vi "Update Offset Dialog.vi"(8 "error in":errorcluster, 10 "Test Result In":T2, 11 "CalCfg File In":T1) -> (0 "error out":errorcluster, 1 "Pass":bool, 2 "Test Result Out":T2, 3 "CalCfg File Out":T1, 4 "String":string)   [LabVIEW 2020, in "GUCalibration2.lvlib"]
uses:
  GUCalibration2.lvlib
  Controls/Test Result.ctl
  Controls/Site Data Element.ctl
  Controls/Site Raw Data Element.ctl
  Controls/Config Data Type.ctl
panel:
  in  "Export Table To CSV":bool
  out "GU Pass Count":string
  out "Result Table":string[][](table)=[["Site_1", "100101", "OS_PS_VDD1_ChA", "0.5", "mA", "0.455881", "0.00", "0.1", "0.2", "0.3", "0.022", ""], ["Site_1", "100102", "OS_PS_VDD1_ChB", "0.5", "uA", "0.467813", "0.00", "0.1", "0.2", "0.3", "0.1317", ""], ["Site_1", "100103", "OS_PS_VDD2_ChB", "0.5", "A", "0.448013", "0.00", "0.1", "0.2", "0.3", "0.0619", ""], ["Site_1", "100104", "OS_PS_SWVDD_ChAB", "0.5", "A", "0.437713", "0.00", "0.1", "0.2", "0.3", "-0.0484", ""], ["Site_1", "100105", "OS_VSS_PPMU_SWCTRL_ChAB", "-0.6", "V", "-0.52606", "0.00", "0.1", "0.2", "0.3", "0.0028", ""], ["Site_1", "100106", "OS_VSS_PPMU_PD_ChAB", "-0.6", "V", "-0.56283", "0.00", "0.1", "0.2", "0.3", "0.0016", ""], ["Site_1", "100107", "OS_VSS_PPMU_BP_ChA", "-0.6", "V", "-0.559845", "0.00", "0.1", "0.2", "0.3", "-0.0132", ""], ["Site_1", "100108", "OS_VSS_PPMU_BP_ChB", "-0.6", "V", "-0.559845", "0.00", "0.1", "0.2", "0.3", "-0.0632", ""], ["Site_1", "200101", "TX_SW_1V8_PD_1V8_BP_0_SWVDD1_ChAB", "0.3", "A", "0.316384", "0.00", "0.1", "0.2", "0.3", "-0.0241", ""], ["Site_1", "200102", "TX_SW_1V8_PD_1V8_BP_0_VDD1_ChA", "0.3", "A", "0.323078", "0.00", "0.1", "0.2", "0.3", "-0.0736", ""], ["Site_1", "200103", "TX_SW_1V8_PD_1V8_BP_0_VDD1_ChB", "0.3", "A", "0.316384", "0.00", "0.1", "0.2", "0.3", "-0.0741", ""], ["Site_1", "200104", "TX_SW_1V8_PD_1V8_BP_0_VDD2_ChB", "0.3", "A", "0.22866", "0.00", "0.1", "0.2", "0.3", "0.0354", ""], ["Site_1", "200105", "RX_SW_0_PD_0_BP_0_VDD1_ChA", "1.85", "A", "1.918991", "0.00", "0.1", "0.2", "0.5", "-0.0378", ""], ["Site_1", "200106", "RX_SW_0_PD_0_BP_0_VDD1_ChB", "1.85", "A", "1.918991", "0.00", "0.1", "0.2", "0.5", "-0.0678", ""], ["Site_1", "200107", "RX_SW_0_PD_0_BP_0_VDD2_ChB", "1.85", "A", "1.908841", "0.00", "0.1", "0.2", "0.5", "0.002", ""], ["Site_1", "200108", "RX_SW_0_PD_0_BP_0_SWVDD_ChAB", "1.85", "A", "1.980908", "0.00", "0.1", "0.2", "0.5", "-0.0686", ""], ["Site_0", "100101", "OS_PS_VDD1_ChA", "0.5", "mA", "0.412485", "0.00", "0.1", "0.2", "0.3", "-0.0147", ""], ["Site_0", "100102", "OS_PS_VDD1_ChB", "0.5", "uA", "0.492041", "0.00", "0.1", "0.2", "0.3", "0.0654", ""], ["Site_0", "100103", "OS_PS_VDD2_ChB", "0.5", "A", "0.481841", "0.00", "0.1", "0.2", "0.3", "0.0052", ""], ["Site_0", "100104", "OS_PS_SWVDD_ChAB", "0.5", "A", "0.471841", "0.00", "0.1", "0.2", "0.3", "-0.1048", ""], ["Site_0", "100105", "OS_VSS_PPMU_SWCTRL_ChAB", "-0.6", "V", "-0.636918", "0.00", "0.1", "0.2", "0.3", "-0.0902", ""], ["Site_0", "100106", "OS_VSS_PPMU_PD_ChAB", "-0.6", "V", "-0.706583", "0.00", "0.1", "0.2", "0.3", "-0.036", ""], ["Site_0", "100107", "OS_VSS_PPMU_BP_ChA", "-0.6", "V", "-0.744575", "0.00", "0.1", "0.2", "0.3", "-0.0387", ""], ["Site_0", "100108", "OS_VSS_PPMU_BP_ChB", "-0.6", "V", "-0.715075", "0.00", "0.1", "0.2", "0.3", "-0.0592", ""], ["Site_0", "200101", "TX_SW_1V8_PD_1V8_BP_0_SWVDD1_ChAB", "0.3", "A", "0.355752", "0.00", "0.1", "0.2", "0.3", "0.0175", ""], ["Site_0", "200102", "TX_SW_1V8_PD_1V8_BP_0_VDD1_ChA", "0.3", "A", "0.363553", "0.00", "0.1", "0.2", "0.3", "-0.03", ""], ["Site_0", "200103", "TX_SW_1V8_PD_1V8_BP_0_VDD1_ChB", "0.3", "A", "0.248228", "0.00", "0.1", "0.2", "0.3", "-0.0428", ""], ["Site_0", "200104", "TX_SW_1V8_PD_1V8_BP_0_VDD2_ChB", "0.3", "A", "0.237628", "0.00", "0.1", "0.2", "0.3", "0.0466", ""], ["Site_0", "200105", "RX_SW_0_PD_0_BP_0_VDD1_ChA", "1.85", "A", "1.71837", "0.00", "0.1", "0.2", "0.5", "0.0158", ""], ["Site_0", "200106", "RX_SW_0_PD_0_BP_0_VDD1_ChB", "1.85", "A", "1.71837", "0.00", "0.1", "0.2", "0.5", "-0.0142", ""], ["Site_0", "200107", "RX_SW_0_PD_0_BP_0_VDD2_ChB", "1.85", "A", "1.75781", "0.00", "0.1", "0.2", "0.5", "0.0696", ""], ["Site_0", "200108", "RX_SW_0_PD_0_BP_0_SWVDD_ChAB", "1.85", "A", "1.591898", "0.00", "0.1", "0.2", "0.5", "-0.1017", ""]]
  out "Update Execute?":bool
  out "Info Disp":string
  in  "Update Offset":bool
  in  "Cancel":bool
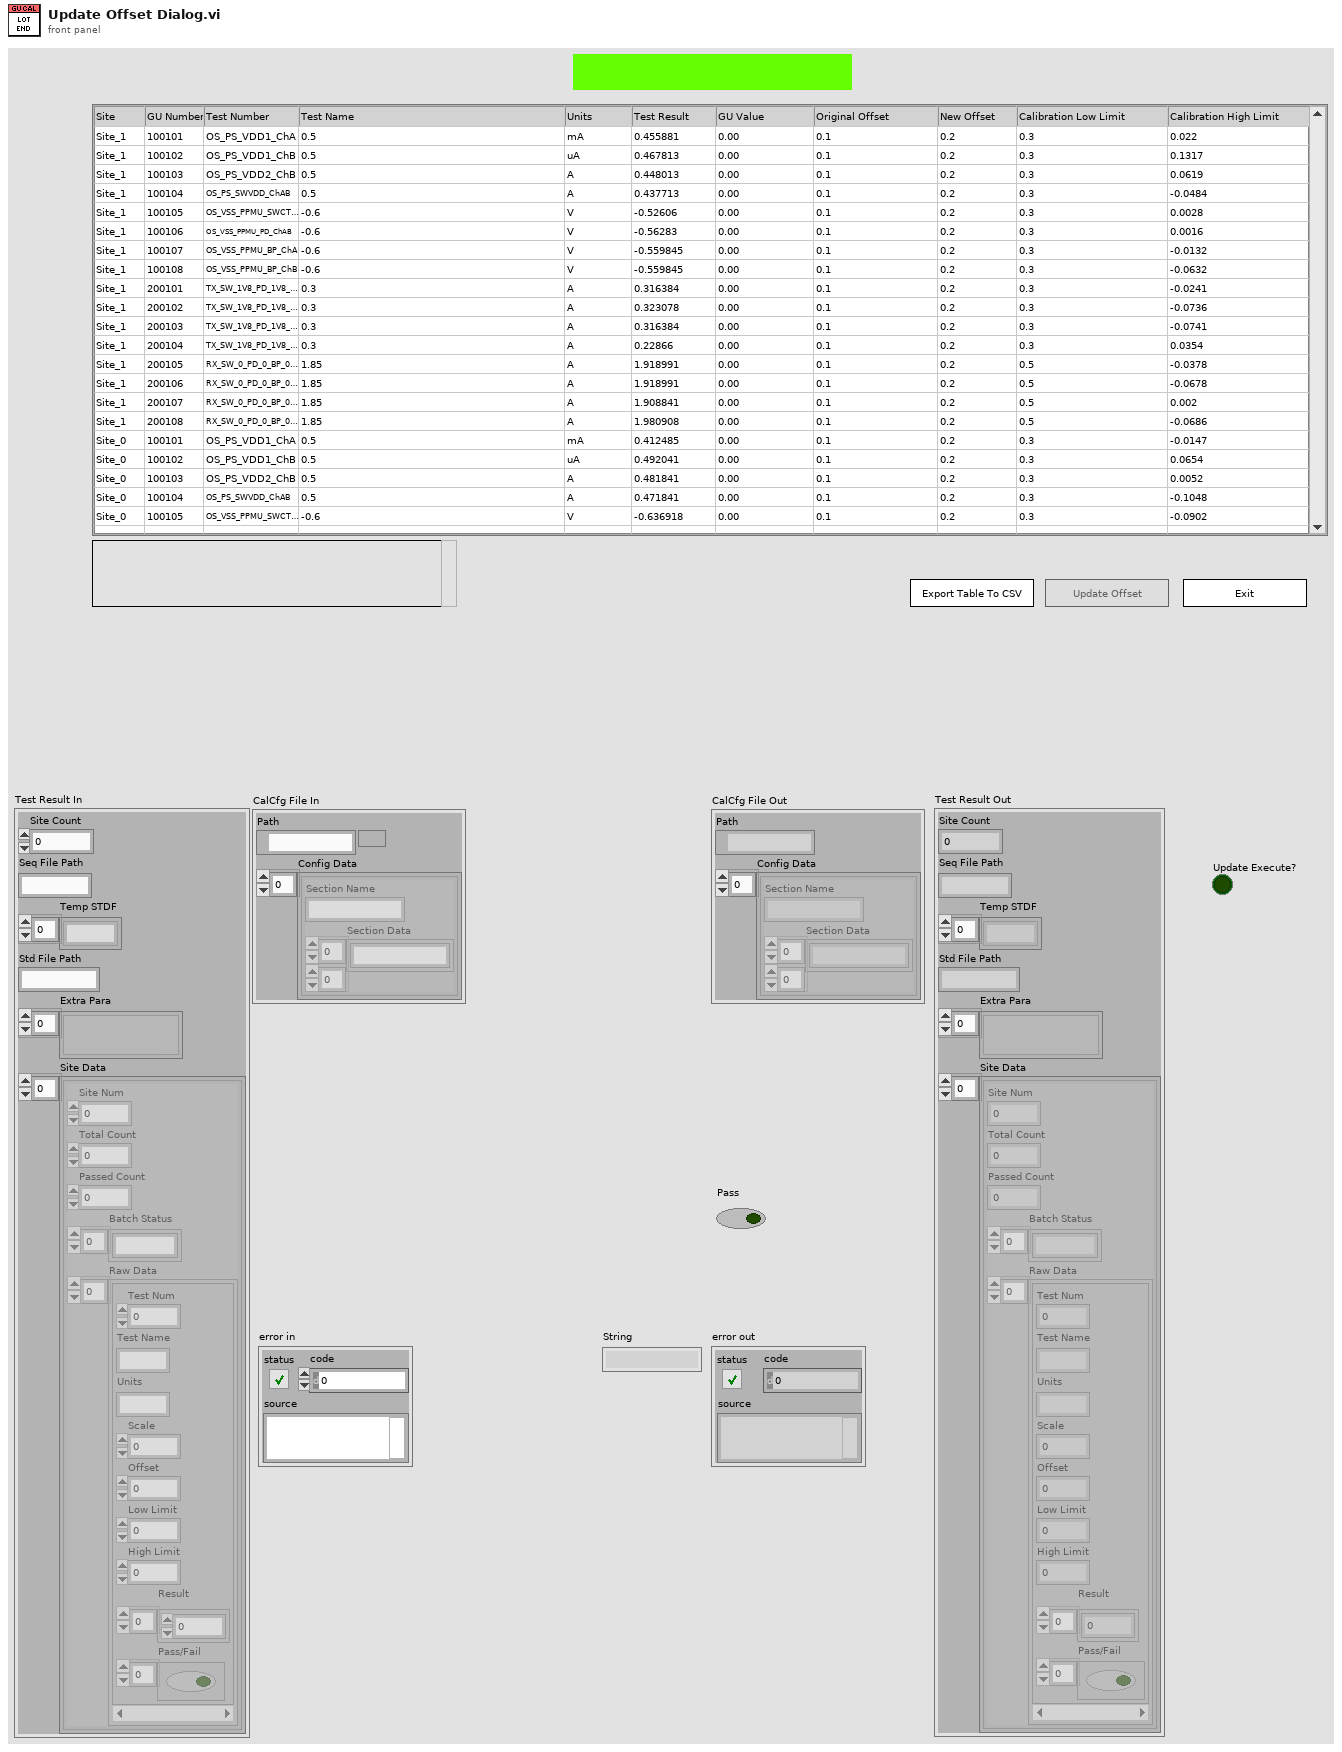
[diagram p1: front panel]
types:
  T1 = cluster{"Path":path, "Config Data":cluster{"Section Name":string, "Section Data":string[][]}[]}
  T2 = typedef "GUCalibration2.lvlib/Test Result.ctl" = cluster{"Site Count":i32, "Seq File Path":string, "Temp STDF":string[], "Std File Path":string, "Extra Para":variant[], "Site Data":T3[]}
  T3 = typedef "GUCalibration2.lvlib/Site Data Element.ctl" = cluster{"Site Num":i32, "Total Count":i32, "Passed Count":i32, "Batch Status":string[], "Raw Data":T4[]}
  T4 = typedef "GUCalibration2.lvlib/Site Raw Data Element.ctl" = cluster{"Test Num":u32, "Test Name":string, "Units":string, "Scale":i8, "Offset":dbl, "Low Limit":dbl, "High Limit":dbl, "Result":dbl[], "Pass/Fail":bool[]}
  T5 = typedef "GUCalibration2.lvlib/Config Data Type.ctl" = cluster{"Cal Type":i32, "Curr Batch Index":i32, "Loop Count Per GU":i32, "Min Num of Pass GUs Per Site":i32, "Is Calibration":bool, "Batch Iteration Done":bool, "Cal Abort":bool, "Update Offset":bool, "Cal Check Pass":bool, "Cal End":bool, "Enabled Site":i32[], "GU Selected":i32[], "All Available GU":i32[], "GU Arrange":i32[][], "Batch Test Count":i32[][], "Batch Test Result":string[][], "Curr Batch":i32[], "Curr Batch Test Count":i32[], "Curr Batch Target Count":i32[], "Curr Batch Test Result":string[]}
  T6 = cluster{"Result Table":refnum<vi>, "Error":errorcluster, "Exit":bool, "CorrOffset File":cluster{"File Path":path, "Backup File Path":path, "Offset Data":cluster{"Section Name":string, "Section Data":string[][]}[]}, "Calibration Cfg File":cluster{"Path":path, "Config Data":cluster{"Section Name":string, "Section Data":string[][]}[]}, "Test Result":T2, "Col Header":string[], "Data":string[][], "Update OK":bool, "Click Update":bool, "Limit Status":cluster{"Check Limit":bool[], "Cal Limit":bool[], "Cal GU Pass":bool[][], "Check GU Pass":bool[][], "Site Num":i32[], "GU Num":string[][]}, "IsCalibration":bool, "Info Disp":refnum<vi>, "CalType":i32, "Return String":string, "Final Offset":cluster{"Offset Info":cluster{"Site Number":string, "Test Number":string, "Units":string}[][], "Offset Value":string[][]}, "Cal Runtime Cfg":T5, "GU Pass Count Disp":refnum<vi>}
  T7 = cluster{"Section Name":string, "Section Data":string[][]}[]
  T8 = enum8{"Enabled", "Disabled", "Disabled and Grayed Out"}
  T9 = cluster{"File Path":path, "Backup File Path":path, "Offset Data":cluster{"Section Name":string, "Section Data":string[][]}[]}
  T10 = cluster{"Check Limit":bool[], "Cal Limit":bool[], "Cal GU Pass":bool[][], "Check GU Pass":bool[][], "Site Num":i32[], "GU Num":string[][]}
  T11 = cluster{"Offset Info":cluster{"Site Number":string, "Test Number":string, "Units":string}[][], "Offset Value":string[][]}
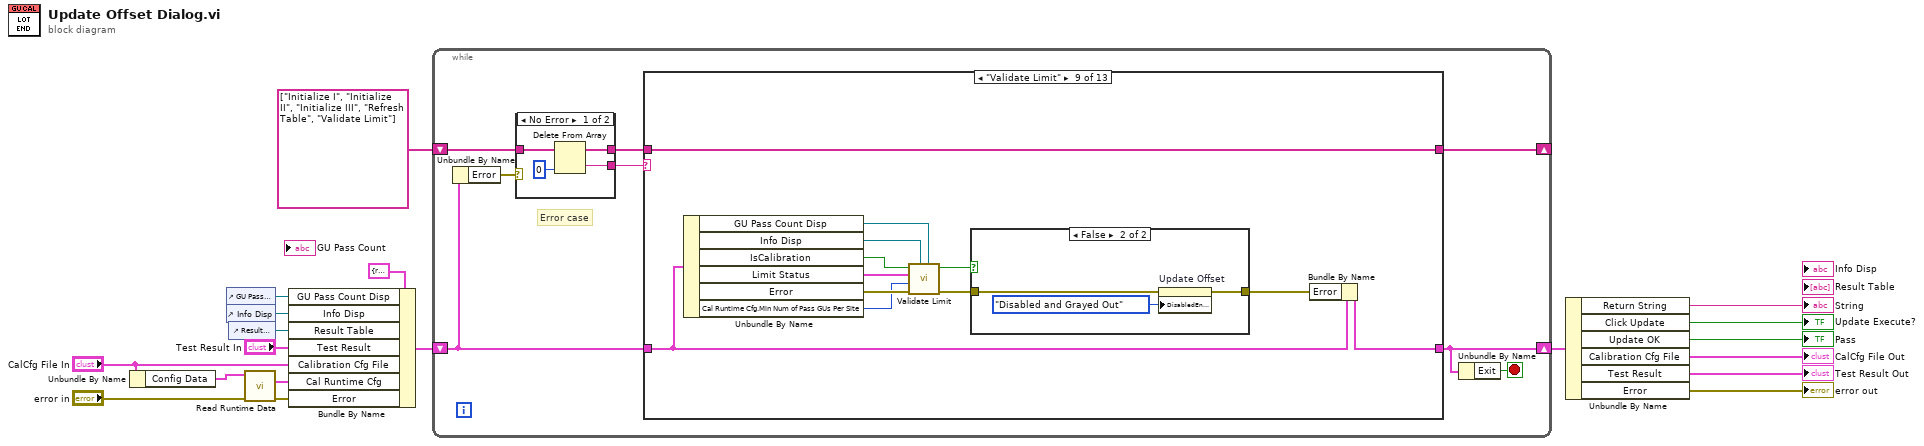
[diagram p0: block diagram]
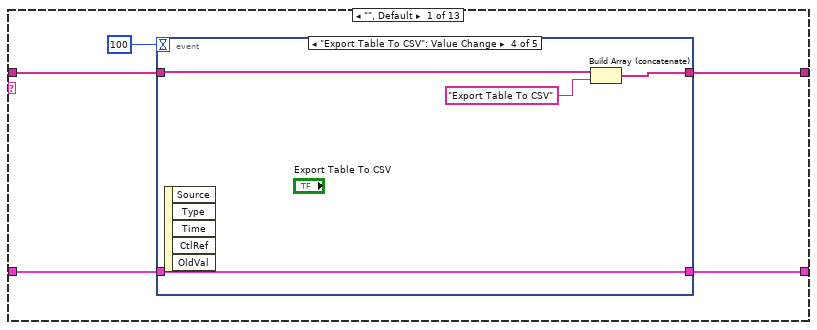
[diagram p2: hidden frame]
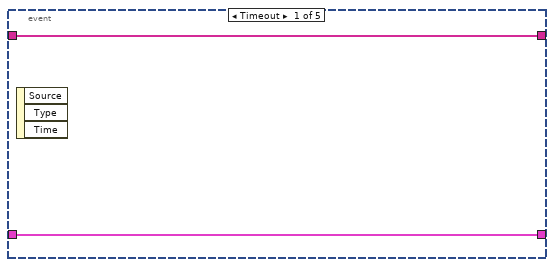
[diagram p3: hidden frame]
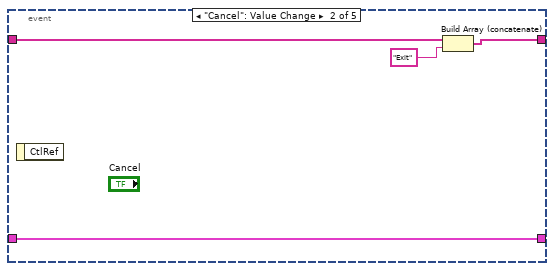
[diagram p4: hidden frame]
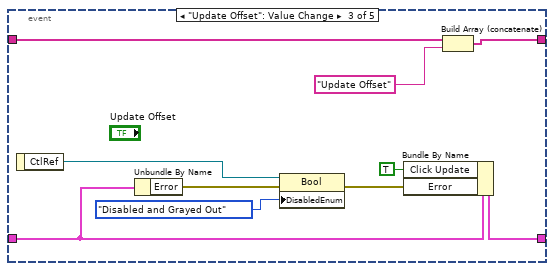
[diagram p5: hidden frame]
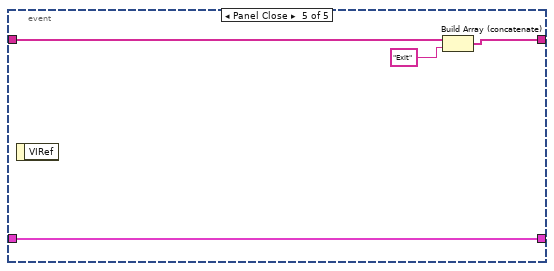
[diagram p6: hidden frame]
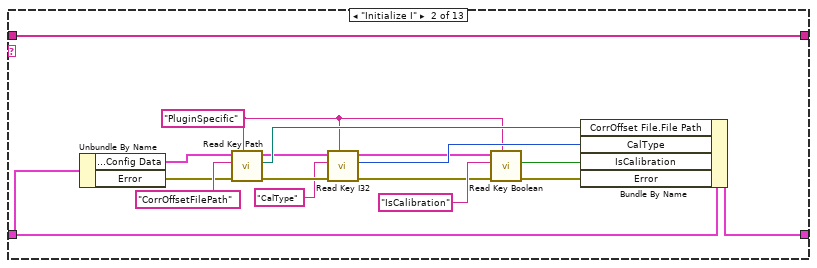
[diagram p7: hidden frame]
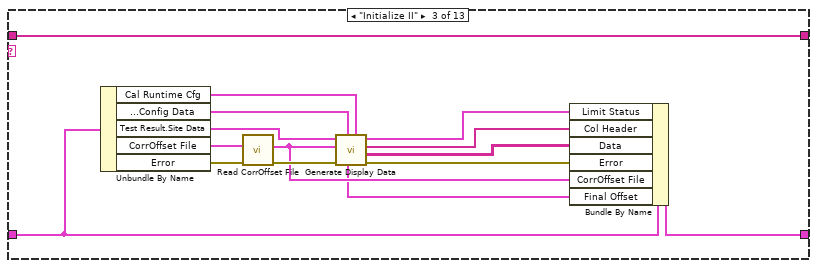
[diagram p8: hidden frame]
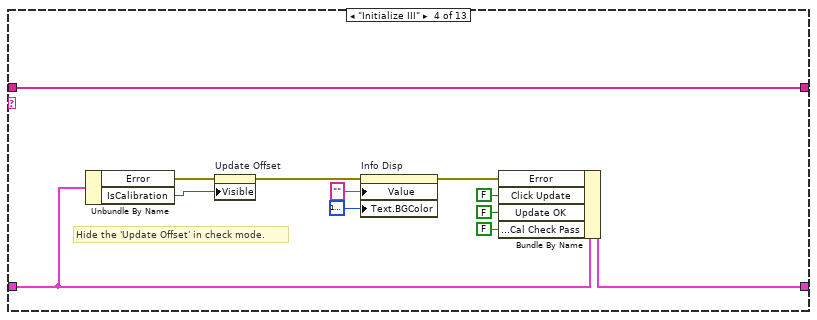
[diagram p9: hidden frame]
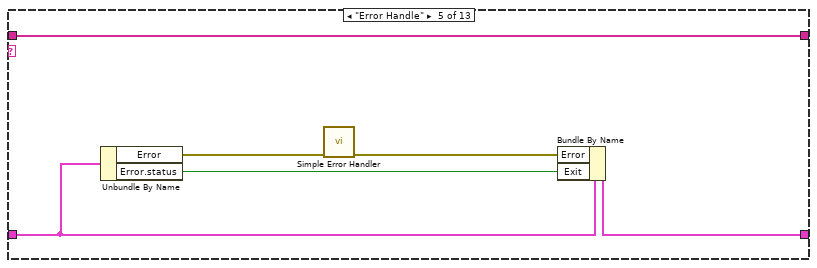
[diagram p10: hidden frame]
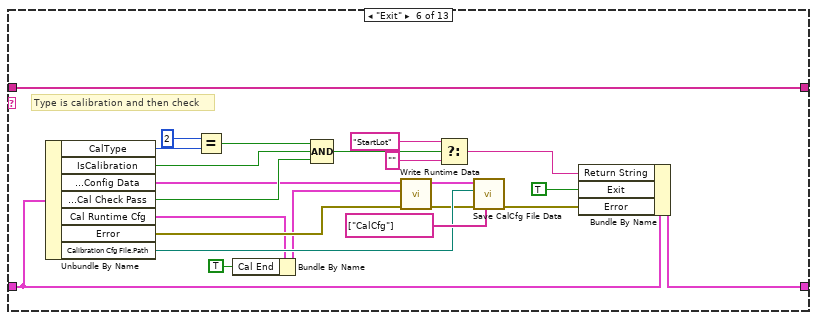
[diagram p11: hidden frame]
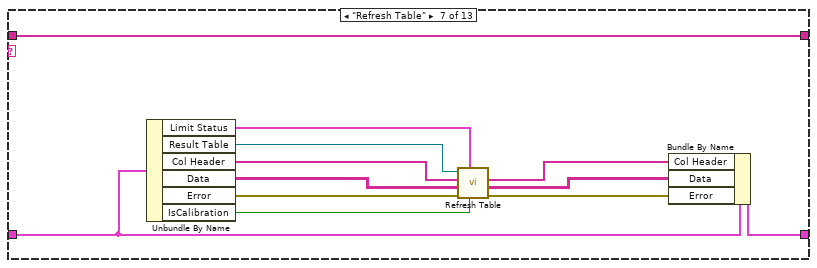
[diagram p12: hidden frame]
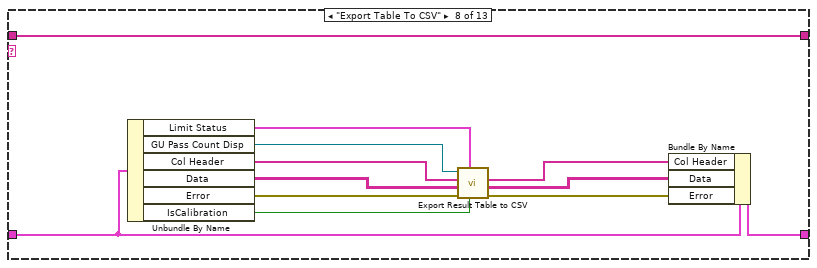
[diagram p13: hidden frame]
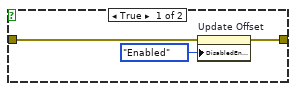
[diagram p14: hidden frame]
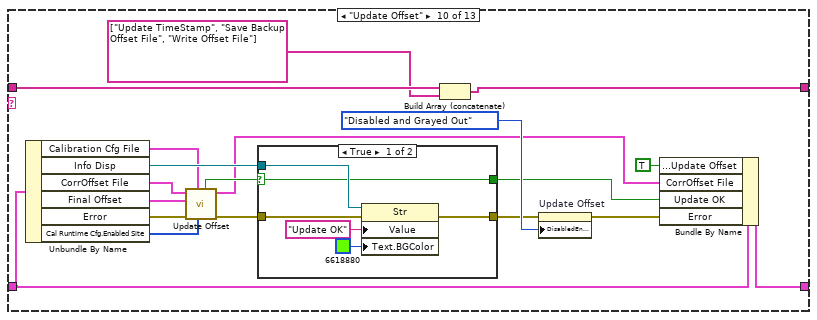
[diagram p15: hidden frame]
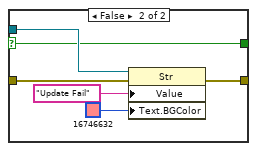
[diagram p16: hidden frame]
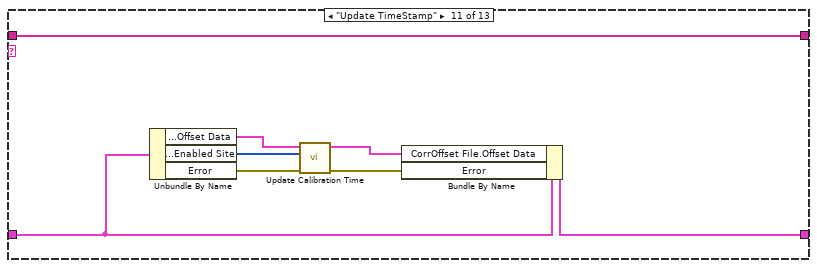
[diagram p17: hidden frame]
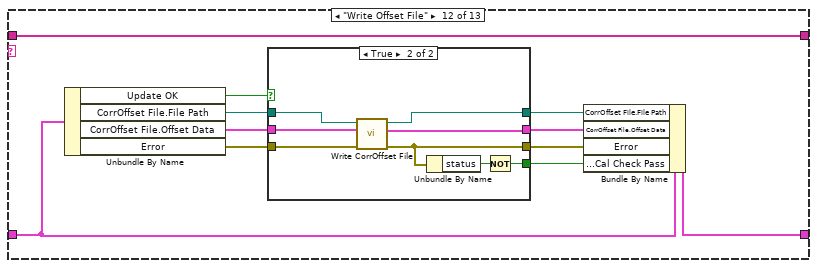
[diagram p18: hidden frame]
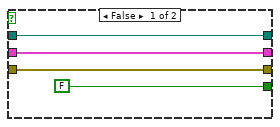
[diagram p19: hidden frame]
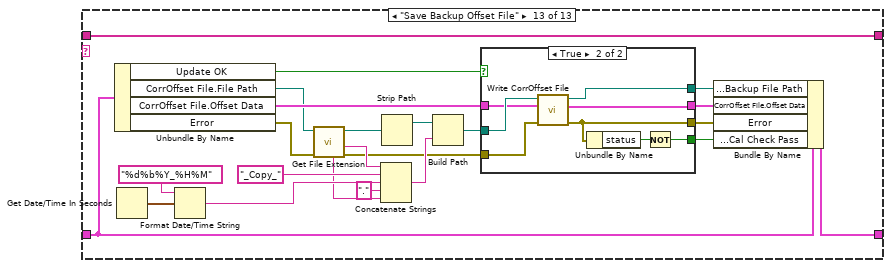
[diagram p20: hidden frame]
diagram:
  n1 = Unbundle By Name("CalCfg File In") -> ("Config Data"=w10:T7)
  n2 = control-ref of="GU Pass Count"() -> (w1:refnum<vi>)
  n3 = control-ref of="Info Disp"() -> (w13:refnum<vi>)
  n4 = control-ref of="Result Table"() -> (w12:refnum<vi>)
  n5 = call "Read Runtime Data.vi"("error in"="error in", "Config File Data In"=w10) -> ("error out"=w8:errorcluster, "Runtime Data Out"=w7:T5)  [unwired: 7 in, 1 out]
  n6 = Bundle By Name(cluster=T6 {"Result Table"=refnum, "Error"={"status"=FALSE, "code"=0, "source"=""}, "Exit"=FALSE, "CorrOffset File"={"File Path"=path "", "Backup File Path"=path "", "Offset Data"=[]}, "Calibration Cfg File"={"Path"=path "", "Config Data"=[]}, "Test Result"={"Site Count"=0, "Seq File Path"="", "Temp STDF"=[], "Std File Path"="", "Extra Para"=[], "Site Data"=[]}, "Col Header"=[], "Data"=[], "Update OK"=FALSE, "Click Update"=FALSE, "Limit Status"={"Check Limit"=[TRUE, TRUE, TRUE, TRUE, TRUE, TRUE, TRUE, TRUE, TRUE, TRUE, TRUE, TRUE, TRUE, TRUE, TRUE, TRUE, TRUE, TRUE, TRUE, TRUE, TRUE, TRUE, TRUE, TRUE], "Cal Limit"=[TRUE, TRUE, TRUE, TRUE, TRUE, TRUE, TRUE, TRUE, TRUE, TRUE, TRUE, TRUE, TRUE, TRUE, TRUE, TRUE, TRUE, TRUE, TRUE, TRUE, TRUE, TRUE, TRUE, TRUE], "Cal GU Pass"=[], "Check GU Pass"=[], "Site Num"=[], "GU Num"=[]}, "IsCalibration"=FALSE, "Info Disp"=refnum, "CalType"=0, "Return String"="", "Final Offset"={"Offset Info"=[], "Offset Value"=[]}, "Cal Runtime Cfg"={"Cal Type"=0, "Curr Batch Index"=0, "Loop Count Per GU"=0, "Min Num of Pass GUs Per Site"=0, "Is Calibration"=FALSE, "Batch Iteration Done"=FALSE, "Cal Abort"=FALSE, "Update Offset"=FALSE, "Cal Check Pass"=FALSE, "Cal End"=FALSE, "Enabled Site"=[], "GU Selected"=[], "All Available GU"=[], "GU Arrange"=[], "Batch Test Count"=[], "Batch Test Result"=[], "Curr Batch"=[], "Curr Batch Test Count"=[], "Curr Batch Target Count"=[], "Curr Batch Test Result"=[]}, "GU Pass Count Disp"=refnum} ("Temp Variables"), "GU Pass Count Disp"=w1, "Info Disp"=w13, "Result Table"=w12, "Test Result"="Test Result In", "Calibration Cfg File"="CalCfg File In", "Cal Runtime Cfg"=w7, "Error"=w8) -> (w3:T6)
  n7 = while {
    shift-right: [w26] -> w6
    shift-left: w3 -> [w27]
    shift-right: [w20] -> _
    shift-left: string[] ["Initialize I", "Initialize II", "Initialize III", "Refresh Table", "Validate Limit"] ("Array") -> [w23]
    stop <- w25 stop-if-true
    # "Error case"
    n8 = Unbundle By Name(w27) -> ("Error"=w24:errorcluster)
    n9 = case shown="No Error" w24 {
      tunnel: w23 -> [w272 w274]
      tunnel: [w271 w274] -> w22
      tunnel: [w270 "Error Handle" ("String")] -> w21
      frame No Error {
        n10 = Delete From Array(array=w272, index=0) -> (deleted portion=w270:string, array with subset deleted=w271:string[])  [unwired: 1 in]
      }
      frame Error {
      }
    }
    n11 = case shown="\"Validate Limit\"" w21 {
      tunnel: w27 -> [w32 w73 w88 w93 w104 w114 w139 w151 w163 w189 w209 w219 w254]
      tunnel: [w31 w72 w87 w99 w105 w115 w140 w152 w164 w190 w210 w220 w255] -> w26
      tunnel: w22 -> [w30 w58 w86 w100 w106 w129 w141 w153 w165 w188 w208 w221 w256]
      tunnel: [w29 w58 w86 w100 w106 w129 w141 w153 w165 w187 w208 w221 w256] -> w20
      frame "", Default {
        n12 = event shown="[3] \"Export Table To CSV\": Value Change" {
          selector: _ -> [_ _ _ _ _]
          dyn-events: _ -> [_ _ _ _ _]
          timeout: 100 -> [_ _ _ _ _]
          tunnel: w32 -> [w34 w35 w44 w52 w53]
          tunnel: [w34 w35 w46 w52 w53] -> w31
          tunnel: w30 -> [w33 w38 w48 w50 w56]
          tunnel: [w33 w37 w47 w49 w55] -> w29
          event Timeout {
            n13 = event-data() -> ()  [unwired: 1 in, 3 out]
          }
          event "Cancel": Value Change {
            n14 = event-data() -> ()  [unwired: 1 in, 1 out]
            n15 = Build Array (concatenate)(w38, "Exit" ("String")) -> (w37:string[])
          }
          event "Update Offset": Value Change {
            n16 = event-data() -> ("CtlRef"=w42:refnum<vi>)  [unwired: 1 in]
            n17 = Unbundle By Name(w44) -> ("Error"=w43:errorcluster)
            n18 = property class="Bool"(reference=w42, error in=w43, "DisabledEnum"=T8."Disabled and Grayed Out" ("Disabled")) -> (error out=w40:errorcluster)  [unwired: 1 out]
            n19 = Bundle By Name(cluster=w44, "Click Update"=TRUE, "Error"=w40) -> (w46:T6)
            n20 = Build Array (concatenate)(w48, "Update Offset" ("String")) -> (w47:string[])
          }
          event "Export Table To CSV": Value Change {
            n21 = event-data() -> ()  [unwired: 1 in, 5 out]
            n22 = Build Array (concatenate)(w50, "Export Table To CSV" ("String")) -> (w49:string[])
          }
          event Panel Close {
            n23 = event-data() -> ()  [unwired: 1 in, 1 out]
            n24 = Build Array (concatenate)(w56, "Exit" ("String")) -> (w55:string[])
          }
        }
      }
      frame "Initialize I" {
        w59 = "PluginSpecific" ("Section Name")
        n25 = Unbundle By Name(w73) -> ("Calibration Cfg File.Config Data"=w66:T7, "Error"=w65:errorcluster)
        n26 = call "Read Key Path.vi"("Section Name"=w59, "error in (no error)"=w65, "Key Names"="CorrOffsetFilePath" ("Section Name"), "Config Data"=w66) -> ("error out"=w69:errorcluster, "Key Value out"=w70:path, "Config Data dup"=w68:T7)  [unwired: 3 in, 2 out]
        n27 = call "Read Key I32.vi"("Section Name"=w59, "error in (no error)"=w69, "Key Names"="CalType" ("Section Name"), "Config Data"=w68) -> ("error out"=w62:errorcluster, "Key Value out"=w64:i32, "Config Data dup"=w61:T7)  [unwired: 3 in, 2 out]
        n28 = call "Read Key Boolean.vi"("Section Name"=w59, "error in (no error)"=w62, "Key Names"="IsCalibration" ("Section Name"), "Config Data"=w61) -> ("error out"=w57:errorcluster, "Key Value out"=w60:bool)  [unwired: 3 in, 3 out]
        n29 = Bundle By Name(cluster=w73, "CorrOffset File.File Path"=w70, "CalType"=w64, "IsCalibration"=w60, "Error"=w57) -> (w72:T6)
      }
      frame "Initialize II" {
        n30 = Unbundle By Name(w88) -> ("Cal Runtime Cfg"=w76:T5, "Calibration Cfg File.Config Data"=w74:T7, "Test Result.Site Data"=w75:T3[], "CorrOffset File"=w80:T9, "Error"=w82:errorcluster)
        n31 = call "Read CorrOffset File.vi"("error in"=w82, "CorrOffset File In"=w80) -> ("error out"=w81:errorcluster, "CorrOffset File Out"=w79:T9)  [unwired: 8 in]
        n32 = call "Generate Display Data.vi"("Cal Runtime Cfg"=w76, "Config Data"=w74, "error in"=w81, "CorrOffset File In"=w79, "Site Data"=w75) -> ("error out"=w83:errorcluster, "Data String"=w84:string[][], "Col Header String"=w85:string[], "Limit Status"=w77:T10, "Final Offset"=w78:T11)  [unwired: 2 in]
        n33 = Bundle By Name(cluster=w88, "Limit Status"=w77, "Col Header"=w85, "Data"=w84, "Error"=w83, "CorrOffset File"=w79, "Final Offset"=w78) -> (w87:T6)
      }
      frame "Initialize III" {
        # "Hide the 'Update Offset' in check mode."
        n34 = Unbundle By Name(w93) -> ("Error"=w91:errorcluster, "IsCalibration"=w90:bool)
        n35 = property on="Update Offset" class="Bool"(error in=w91, "Visible"=w90) -> (error out=w89:errorcluster)  [unwired: 1 in, 1 out]
        n36 = property on="Info Disp" class="Str"(error in=w89, "Value"="" ("Info Disp"), "Text.BGColor"=u32 16777225) -> (error out=w96:errorcluster)  [unwired: 1 in, 1 out]
        n37 = Bundle By Name(cluster=w93, "Error"=w96, "Click Update"=FALSE, "Update OK"=FALSE, "Cal Runtime Cfg.Cal Check Pass"=FALSE ("CompCheckPass")) -> (w99:T6)
      }
      frame "Error Handle" {
        n38 = Unbundle By Name(w104) -> ("Error"=w102:errorcluster, "Error.status"=w103:bool)
        n39 = call <vilib>:"Simple Error Handler.vi"("error in (no error)"=w102) -> ("error out"=w101:errorcluster)  [unwired: 4 in, 4 out]
        n40 = Bundle By Name(cluster=w104, "Error"=w101, "Exit"=w103) -> (w105:T6)
      }
      frame "Exit" {
        # "Type is calibration and then check"
        n41 = Unbundle By Name(w114) -> ("CalType"=w127:i32, "IsCalibration"=w119:bool, "Calibration Cfg File.Config Data"=w112:T7, "Cal Runtime Cfg.Cal Check Pass"=w118:bool, "Cal Runtime Cfg"=w111:T5, "Error"=w113:errorcluster, "Calibration Cfg File.Path"=w120:path)
        n42 = Equal?(x=2, y=w127) -> (x = y?=w125:bool)
        n43 = Bundle By Name(cluster=w111, "Cal End"=TRUE) -> (w108:T5)
        n44 = Compound Arithmetic op=AND(w125, w119, w118) -> (w117:bool)
        n45 = call "Write Runtime Data.vi"("error in"=w113, "Runtime Data In"=w108, "Config File Data In"=w112) -> ("error out"=w110:errorcluster, "Config Data Out"=w109:T7)  [unwired: 6 in, 1 out]
        n46 = Select(t="StartLot" ("String"), s=w117, f="") -> (s? t:f=w116:string)
        n47 = call "Save CalCfg File Data.vi"("Matric Section"=string[] ["CalCfg"], "error in"=w110, "File Path"=w120, "Config Data"=w109) -> ("error out"=w121:errorcluster)  [unwired: 7 in]
        n48 = Bundle By Name(cluster=w114, "Return String"=w116, "Exit"=TRUE, "Error"=w121) -> (w115:T6)
      }
      frame "Refresh Table" {
        n49 = Unbundle By Name(w139) -> ("Limit Status"=w130:T10, "Result Table"=w137:refnum<vi>, "Col Header"=w136:string[], "Data"=w135:string[][], "Error"=w138:errorcluster, "IsCalibration"=w131:bool)
        n50 = call "Refresh Table.vi"("IsCalibration"=w131, "Limit Status"=w130, "error in"=w138, "Data String"=w135, "Col Header String"=w136, "Result Table"=w137) -> ("error out"=w134:errorcluster, "Data String dup"=w132:string[][], "Col Header String dup"=w133:string[])  [unwired: 2 in, 1 out]
        n51 = Bundle By Name(cluster=w139, "Col Header"=w133, "Data"=w132, "Error"=w134) -> (w140:T6)
      }
      frame "Export Table To CSV" {
        n52 = Unbundle By Name(w151) -> ("Limit Status"=w143:T10, "GU Pass Count Disp"=w149:refnum<vi>, "Col Header"=w148:string[], "Data"=w147:string[][], "Error"=w150:errorcluster, "IsCalibration"=w142:bool)
        n53 = call "Export Result Table to CSV.vi"("IsCalibration"=w142, "Limit Status"=w143, "error in"=w150, "Data String"=w147, "Col Header String"=w148, "GU Pass Count Indicator"=w149) -> ("error out"=w146:errorcluster, "Data String dup"=w144:string[][], "Col Header String dup"=w145:string[])  [unwired: 3 in]
        n54 = Bundle By Name(cluster=w151, "Col Header"=w145, "Data"=w144, "Error"=w146) -> (w152:T6)
      }
      frame "Validate Limit" {
        n55 = Unbundle By Name(w163) -> ("GU Pass Count Disp"=w154:refnum<vi>, "Info Disp"=w161:refnum<vi>, "IsCalibration"=w158:bool, "Limit Status"=w157:T10, "Error"=w162:errorcluster, "Cal Runtime Cfg.Min Num of Pass GUs Per Site"=w155:i32)
        n56 = call "Validate Limit.vi"("GU Pass Count Disp"=w154, "Info Disp"=w161, "error in"=w162, "Min Pass Num Per Batch"=w155, "Limit Status"=w157, "IsCalibration"=w158) -> ("error out"=w160:errorcluster, "Update Offset"=w156:bool)  [unwired: 4 in]
        n57 = case shown="False" w156 {
          tunnel: w160 -> [w166 w171]
          tunnel: [w167 w169] -> w159
          frame True {
            n58 = property on="Update Offset" class="Bool"(error in=w166, "DisabledEnum"=T8."Enabled" ("Disabled")) -> (error out=w167:errorcluster)  [unwired: 1 in, 1 out]
          }
          frame False {
            n59 = property on="Update Offset" class="Bool"(error in=w171, "DisabledEnum"=T8."Disabled and Grayed Out" ("Disabled")) -> (error out=w169:errorcluster)  [unwired: 1 in, 1 out]
          }
        }
        n60 = Bundle By Name(cluster=w163, "Error"=w159) -> (w164:T6)
      }
      frame "Update Offset" {
        n61 = Unbundle By Name(w189) -> ("Calibration Cfg File"=w175:T1, "Info Disp"=w182:refnum<vi>, "CorrOffset File"=w176:T9, "Final Offset"=w179:T11, "Error"=w184:errorcluster, "Cal Runtime Cfg.Enabled Site"=w174:i32[])
        n62 = call "Update Offset.vi"("Enabled Site"=w174, "Calibration Cfg File"=w175, "error in"=w184, "Final Offset"=w179, "CorrOffset File In"=w176) -> ("error out"=w181:errorcluster, "CorrOffset File Out"=w177:T9, "Update OK"=w180:bool)  [unwired: 4 in]
        n63 = case shown="True" w180 {
          selector: w180 -> [w191 w197]
          tunnel: w181 -> [w192 w202]
          tunnel: [w196 w201] -> w183
          tunnel: w182 -> [w195 w200]
          tunnel: [w191 w197] -> w178
          frame True {
            n64 = property class="Str"(reference=w195, error in=w192, "Value"="Update OK", "Text.BGColor"=u32 6618880) -> (error out=w196:errorcluster)  [unwired: 1 out]
          }
          frame False {
            n65 = property class="Str"(reference=w200, error in=w202, "Value"="Update Fail", "Text.BGColor"=u32 16746632) -> (error out=w201:errorcluster)  [unwired: 1 out]
          }
        }
        n66 = Build Array (concatenate)(w188, string[] ["Update TimeStamp", "Save Backup Offset File", "Write Offset File"] ("Array")) -> (w187:string[])
        n67 = property on="Update Offset" class="Bool"(error in=w183, "DisabledEnum"=T8."Disabled and Grayed Out" ("Disabled")) -> (error out=w185:errorcluster)  [unwired: 1 in, 1 out]
        n68 = Bundle By Name(cluster=w189, "Cal Runtime Cfg.Update Offset"=TRUE, "CorrOffset File"=w177, "Update OK"=w178, "Error"=w185) -> (w190:T6)
      }
      frame "Update TimeStamp" {
        n69 = Unbundle By Name(w209) -> ("CorrOffset File.Offset Data"=w206:T7, "Cal Runtime Cfg.Enabled Site"=w205:i32[], "Error"=w207:errorcluster)
        n70 = call "Update Calibration Time.vi"("error in"=w207, "Update Sites"=w205, "Offset Data"=w206) -> ("error out"=w203:errorcluster, "Offset Data Out"=w204:T7)  [unwired: 7 in]
        n71 = Bundle By Name(cluster=w209, "CorrOffset File.Offset Data"=w204, "Error"=w203) -> (w210:T6)
      }
      frame "Write Offset File" {
        n72 = Unbundle By Name(w219) -> ("Update OK"=w211:bool, "CorrOffset File.File Path"=w216:path, "CorrOffset File.Offset Data"=w213:T7, "Error"=w218:errorcluster)
        n73 = case shown="True" w211 {
          tunnel: w218 -> [w225 w227]
          tunnel: [w225 w233] -> w217
          tunnel: w216 -> [w223 w230]
          tunnel: [FALSE w231] -> w212
          tunnel: w213 -> [w222 w226]
          tunnel: [w223 w229] -> w215
          tunnel: [w222 w228] -> w214
          frame False {
          }
          frame True {
            n74 = call "Write CorrOffset File.vi"("error in"=w227, "Offset Data In"=w226, "File Path In"=w230) -> ("error out"=w233:errorcluster, "Offset Data Out"=w228:T7, "File Path Out"=w229:path)  [unwired: 6 in]
            n75 = Unbundle By Name(w233) -> ("status"=w232:bool)
            n76 = Not(x=w232) -> (.not. x?=w231:bool)
          }
        }
        n77 = Bundle By Name(cluster=w219, "CorrOffset File.File Path"=w215, "CorrOffset File.Offset Data"=w214, "Error"=w217, "Cal Runtime Cfg.Cal Check Pass"=w212) -> (w220:T6)
      }
      frame "Save Backup Offset File" {
        n78 = Unbundle By Name(w254) -> ("Update OK"=w234:bool, "CorrOffset File.File Path"=w244:path, "CorrOffset File.Offset Data"=w252:T7, "Error"=w245:errorcluster)
        n79 = Get Date/Time In Seconds() -> (seconds since 1Jan1904=w248:timestamp)
        n80 = Format Date/Time String(time format string (%c)="%d%b%Y_%H%M", seconds (now)=w248) -> (date/time string=w246:string)  [unwired: 1 in]
        n81 = call <vilib>:"Get File Extension.vi"("error in (no error)"=w245, "file"=w244) -> ("error out"=w236:errorcluster, "filename without extension"=w241:string, "dup file"=w243:path, "unmodified file extension"=w239:string)  [unwired: 5 in, 1 out]
        n82 = Concatenate Strings(w241, "_Copy_" ("time format string (%c)"), w246, "." ("string"), w239) -> (w240:string)
        n83 = Strip Path(path=w243) -> (stripped path=w242:path)  [unwired: 1 out]
        n84 = Build Path(base path=w242, name or relative path=w240) -> (appended path=w237:path)
        n85 = case shown="True" w234 {
          tunnel: w236 -> [w260 w262]
          tunnel: [w260 w268] -> w253
          tunnel: w237 -> [w258 w265]
          tunnel: [FALSE w266] -> w235
          tunnel: w252 -> [w257 w261]
          tunnel: [w258 w264] -> w251
          tunnel: [w257 w263] -> w250
          frame False {
          }
          frame True {
            n86 = call "Write CorrOffset File.vi"("error in"=w262, "Offset Data In"=w261, "File Path In"=w265) -> ("error out"=w268:errorcluster, "Offset Data Out"=w263:T7, "File Path Out"=w264:path)  [unwired: 6 in]
            n87 = Unbundle By Name(w268) -> ("status"=w267:bool)
            n88 = Not(x=w267) -> (.not. x?=w266:bool)
          }
        }
        n89 = Bundle By Name(cluster=w254, "CorrOffset File.Backup File Path"=w251, "CorrOffset File.Offset Data"=w250, "Error"=w253, "Cal Runtime Cfg.Cal Check Pass"=w235) -> (w255:T6)
      }
    }
    n90 = Unbundle By Name(w26) -> ("Exit"=w25:bool)
  }
  n91 = Unbundle By Name(w6) -> ("Return String"=→"String":string, "Click Update"=→"Update Execute?":bool, "Update OK"=→"Pass":bool, "Calibration Cfg File"=→"CalCfg File Out":T1, "Test Result"=→"Test Result Out":T2, "Error"=→"error out":errorcluster)
